vi "DELETEDAQ.PreStartWriteBuffer.vi"(8 "error in (no error)":errorcluster, 11 "Instrument.DAQ in":refnum<class "Instrument.DAQ.lvclass">) -> (0 "error out":errorcluster, 3 "Instrument.DAQ out":refnum<class "Instrument.DAQ.lvclass">)   [LabVIEW 2019]
uses:
  Instrument.DAQ/Instrument.DAQ.lvclass
  Generator/Generator.lvclass
  DAQmx/DAQmx.lvclass
  Generator/typedefs/Sweep.State--enum.ctl
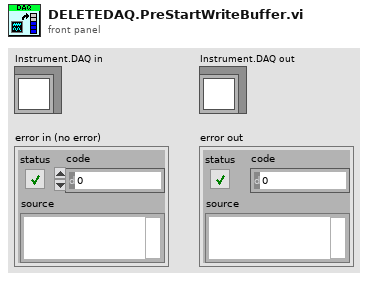
[diagram p1: front panel]
types:
  T1 = typedef "Generator.lvclass/Sweep.State--enum.ctl" = enum16{"idle", "initialize", "wait", "sweep", "stop"}
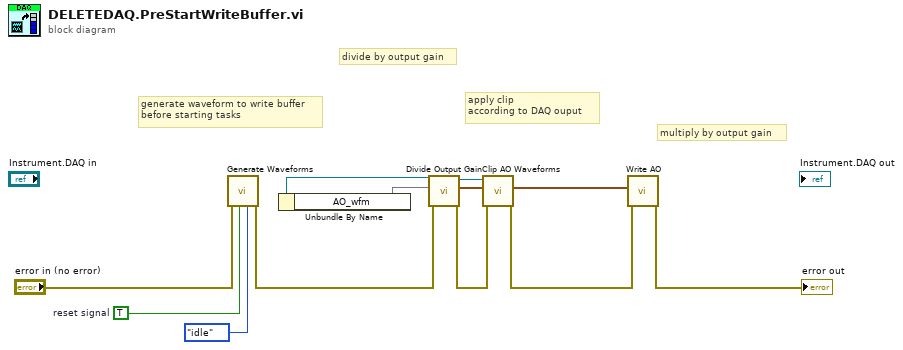
[diagram p0: block diagram]
diagram:
  w3 = TRUE  # reset signal
  # "multiply by output gain"
  # "generate waveform to write buffer\nbefore starting tasks"
  # "apply clip\naccording to DAQ ouput"
  # "divide by output gain"
  n1 = call "Generate Waveforms.vi"("sweep state"=Sweep.State--enum."idle", "Reset Phase?"=w3, "error in (no error)"="error in (no error)") -> ("error out"=w7:errorcluster)  [unwired: 7 in, 1 out]
  n2 = Unbundle By Name(w8) -> ("AO_wfm"=w9)
  n3 = call "Divide Output Gain.vi"("error in (no error)"=w7, "WFM in"=w9) -> ("error out"=w6:errorcluster, "WFM out"=w4:waveform(dbl)[], "Instrument.DAQ out"=w5:refnum<class "Instrument.DAQ.lvclass">, "Instrument.DAQ"=w8:refnum<class "Instrument.DAQ.lvclass">)  [unwired: 6 in]
  n4 = call "Clip AO Waveforms.vi"("error in (no error)"=w6, "AO []"=w4, "Instrument.DAQ in"=w5) -> ("error out"=w12:errorcluster, "Clipped AO []"=w11:waveform(dbl)[])  [unwired: 6 in, 1 out]
  n5 = call "Write AO.vi"("error in (no error)"=w12, "AO []"=w11) -> ("error out"=→"error out":errorcluster)  [unwired: 6 in, 3 out]
